vi "Outlet Convert Temp to Volt.vi"(0 "Model IN":enum16{"Estar Centauro", "GFL"}(ring), 7 "Outlet Temperature":dbl, 11 "Error In":errorcluster) -> (8 "Outlet Voltage":dbl, 15 "Error Out":errorcluster)   [LabVIEW 2021]
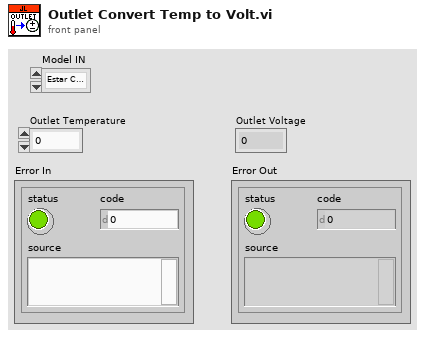
[diagram p1: front panel]
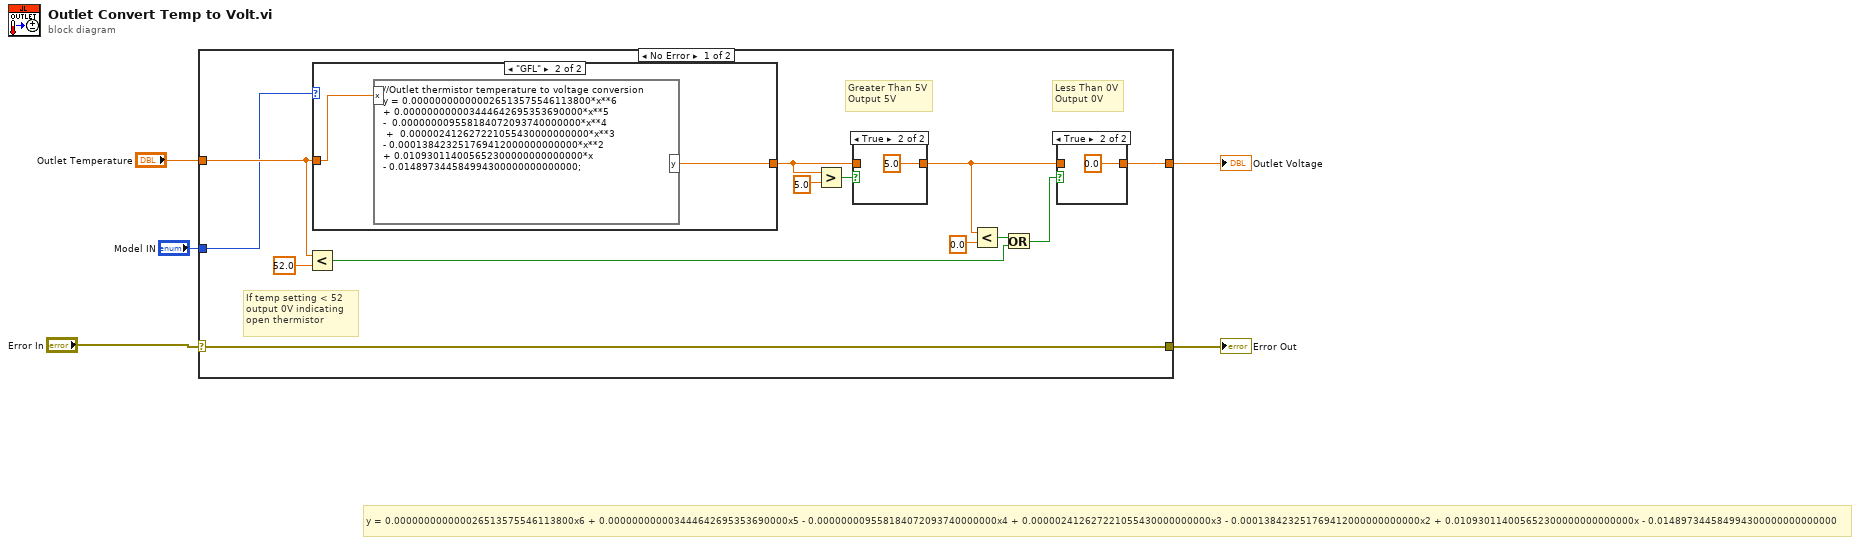
[diagram p0: block diagram]
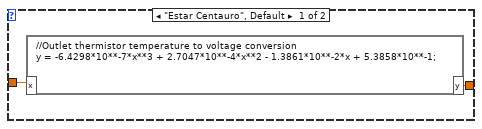
[diagram p2: hidden frame]
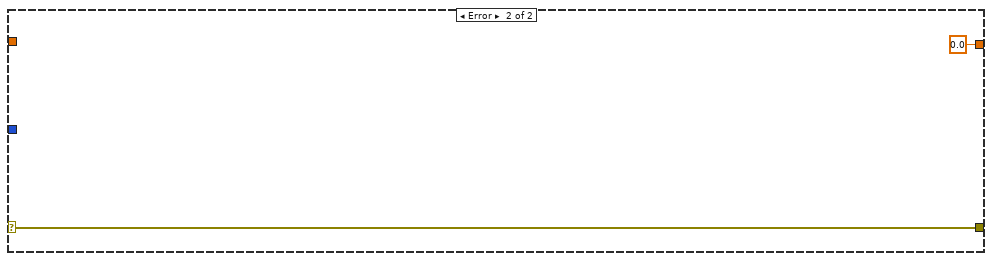
[diagram p5: hidden frame]
diagram:
  # "y = 0.000000000000026513575546113800x6 + 0.000000000003444642695353690000x5 - 0.000000009558184072093740000000x4 + 0.000002412627221055430000000000x3 - 0.000138423251769412000000000000x2 + 0.010930114005652300000000000000x - 0.014897344584994300000000000000"
  n1 = case shown="No Error" "Error In" {
    selector: "Error In" -> [w7 w28]
    tunnel: [w14 0.0 ("y")] -> w5
    tunnel: "Outlet Temperature" -> [w10 _]
    tunnel: [w7 w28] -> w3
    tunnel: "Model IN" -> [w6 _]
    frame No Error {
      # "Less Than 0V\nOutput 0V"
      # "Greater Than 5V\nOutput 5V"
      # "If temp setting < 52 \noutput 0V indicating \nopen thermistor"
      n2 = Less?(x=w10, y=52.0) -> (x < y?=w8:bool)
      n3 = case shown="\"GFL\"" w6 {
        tunnel: [w20 w22] -> w17
        tunnel: w10 -> [w19 w21]
        frame "Estar Centauro", Default {
          n4 = formula code="//Outlet thermistor temperature to voltage conversion\ny = -6.4298*10**-7*x**3 + 2.7047*10**-4*x**2 - 1.3861*10**-2*x + 5.3858*10**-1;"("x"=w19) -> ("y"=w20:dbl)
        }
        frame "GFL" {
          n5 = formula code="//Outlet thermistor temperature to voltage conversion\ny = 0.000000000000026513575546113800*x**6 \n+ 0.000000000003444642695353690000*x**5 \n-  0.000000009558184072093740000000*x**4\n +  0.000002412627221055430000000000*x**3 \n- 0.000138423251769412000000000000*x**2 \n+ 0.010930114005652300000000000000*x \n- 0.014897344584994300000000000000;"("x"=w21) -> ("y"=w22:dbl)
        }
      }
      n6 = Greater?(x=w17, y=5.0) -> (0:w15:bool)
      n7 = case shown="True" w15 {
        tunnel: [w25 5.0 ("y")] -> w13
        tunnel: w17 -> [w25 _]
        frame False {
        }
        frame True {
        }
      }
      n8 = Less?(x=w13, y=0.0) -> (x < y?=w12:bool)
      n9 = Or(x=w12, y=w8) -> (x .or. y?=w11:bool)
      n10 = case shown="True" w11 {
        tunnel: [w23 0.0 ("y")] -> w14
        tunnel: w13 -> [w23 _]
        frame False {
        }
        frame True {
        }
      }
    }
    frame Error {
    }
  }
  "Outlet Voltage" <- w5
  "Error Out" <- w3
